vi "Set file permissions.vi"(7 "Permissions (Writable)":enum16{"Writable", "Read Only"}(ring), 8 "error in":errorcluster, 11 "Path":path) -> (0 "error out":errorcluster, 3 "Path Out":path)   [LabVIEW 2015, in "RT Management.lvlib"]
doc: "Changes the permission of a file to make it writable or read only."
uses:
  RT Management.lvlib
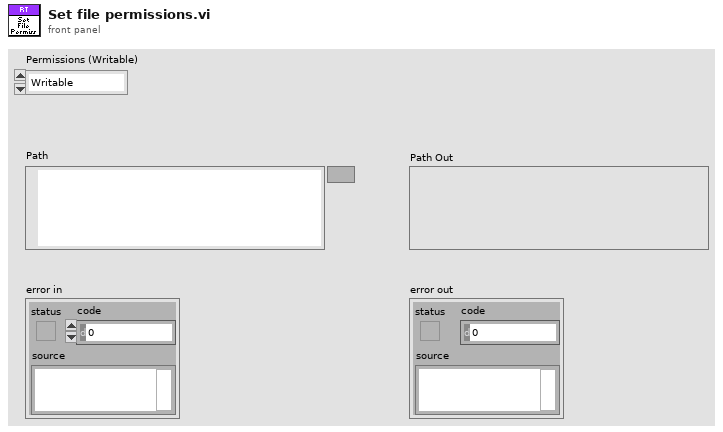
[diagram p1: front panel]
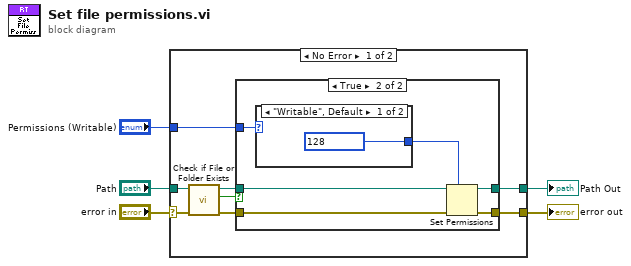
[diagram p0: block diagram]
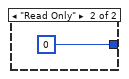
[diagram p3: hidden frame]
diagram:
  n1 = case shown="No Error" "error in" {
    selector: "error in" -> [w10 w25]
    tunnel: [w13 w25] -> w4
    tunnel: "Path" -> [w9 w24]
    tunnel: [w12 w24] -> w2
    tunnel: "Permissions (Writable)" -> [w11 _]
    frame No Error {
      n2 = call <vilib>:"Check if File or Folder Exists.vi"("error in (no error)"=w10, "path"=w9) -> ("error out"=w7:errorcluster, "file or folder exists?"=w6:bool, "dup path"=w8:path)  [unwired: 7 in]
      n3 = case shown="True" w6 {
        tunnel: w7 -> [w15 w21]
        tunnel: [w15 w20] -> w13
        tunnel: w8 -> [w14 w19]
        tunnel: [w14 w18] -> w12
        tunnel: w11 -> [_ w17]
        frame False {
        }
        frame True {
          n4 = case shown="\"Writable\", Default" w17 {
            tunnel: [i16 128 i16 0] -> w16
            frame "Writable", Default {
            }
            frame "Read Only" {
            }
          }
          n5 = Set Permissions(7:w16, 8:w21, 11:w19) -> (0:w20:errorcluster, 3:w18:path)  [unwired: 2 in]
        }
      }
    }
    frame Error {
    }
  }
  "error out" <- w4
  "Path Out" <- w2
